vi "Save Contact.vi"(8 "error in (no error)":errorcluster, 11 "All Lines":T1) -> (0 "error out":errorcluster, 3 "All Lines out":T1)   [LabVIEW 2014, in "Map Data.lvlib"]
doc: "Updates an existing contact or inserts a new contact into the address book data store. Use the ID of an existing contact to update, or an ID of 0 to insert. When inserting, the output cluster will contain the ID of the new contact."
uses:
  Map Data.lvlib
  All-Lines.ctl
  LineCluster.ctl
  LineConnection.ctl
  MapCommand.ctl
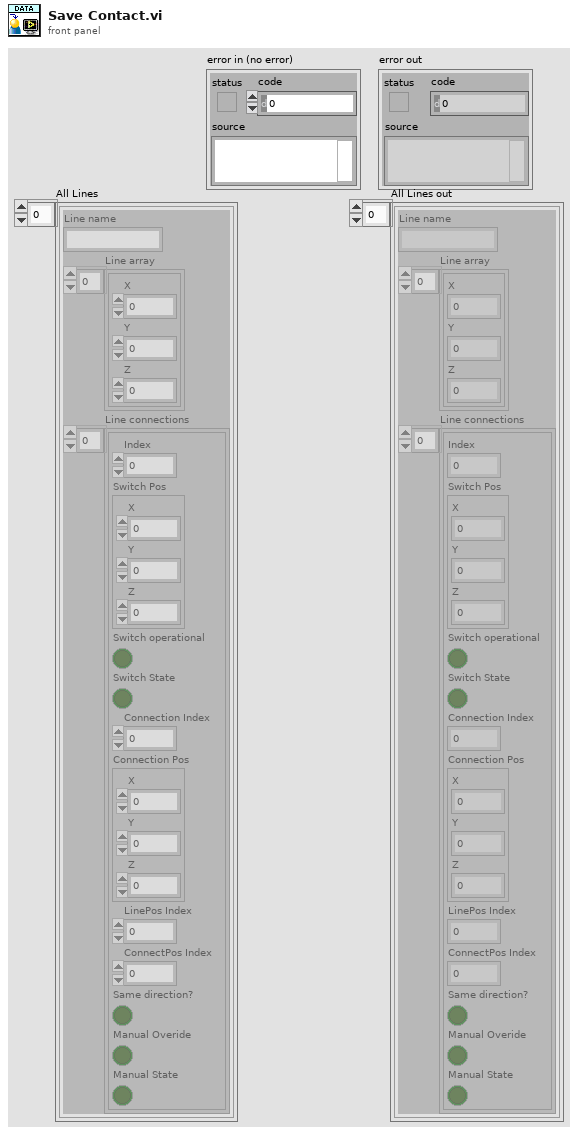
[diagram p1: front panel]
types:
  T1 = typedef "Map Data.lvlib/All-Lines.ctl" = T2[]
  T2 = typedef "Map Data.lvlib/LineCluster.ctl" = cluster{"Line name":string, "Line array":cluster{"X":dbl, "Y":dbl, "Z":dbl}[], "Line connections":T3[]}
  T3 = typedef "Map Data.lvlib/LineConnection.ctl" = cluster{"Index":i32, "Switch Pos":cluster{"X":dbl, "Y":dbl, "Z":dbl}, "Switch operational":bool, "Switch State":bool, "Connection Index":i32, "Connection Pos":cluster{"X":dbl, "Y":dbl, "Z":dbl}, "LinePos Index":i32, "ConnectPos Index":i32, "Same direction?":bool, "Manual Overide":bool, "Manual State":bool}
  T4 = typedef "Map Data.lvlib/MapCommand.ctl" = enum16{"Load", "Update Cursor", "Save", "Get All Data", "Get Single Data", "Set Single Data", "Delete All", "Remove Single Data", "Set Favorite Status", "Is Data Modified", "Import Data"}
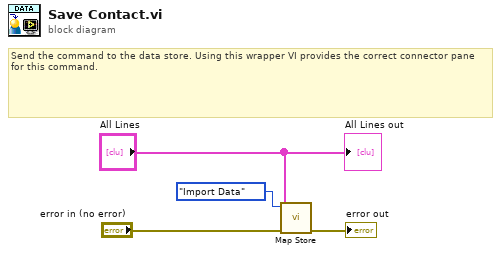
[diagram p0: block diagram]
diagram:
  # "Send the command to the data store. Using this wrapper VI provides the correct connector pane for this command."
  n1 = call "Map Store.vi"("error in (no error)"="error in (no error)", "All Lines"="All Lines", "Command"=MapCommand."Import Data") -> ("error out"=→"error out":errorcluster)  [unwired: 5 in, 3 out]
  "All Lines out" <- "All Lines"
